vi "doDFSM_Alive.vi"(0 "HGF_DeviceBase":refnum<class "HGF_DeviceBase.lvclass">, 3 "DFSM_Internals in":T1, 5 "error in (no error)":errorcluster) -> (14 "dup HGF_DeviceBase":refnum<class "HGF_DeviceBase.lvclass">, 17 "DFSM_Internals out":T1, 19 "error out":errorcluster)   [LabVIEW 2014, in "HGF_DeviceBaseClasses.lvlib" / "HGF_DeviceBase.lvclass"]
doc: "This VI performs <B>do</B> action of DeviceFSM.Alive.\n\n<b>Hint:</b> This is a dynamic dispatch VI to be implemented by child classes."
uses:
  HGF_DeviceBase.lvclass
  HGF_StateCharts/HGF_DeviceFSM/HGF_DeviceFSM_Internals.ctl
  HGF_DeviceBaseClasses.lvlib
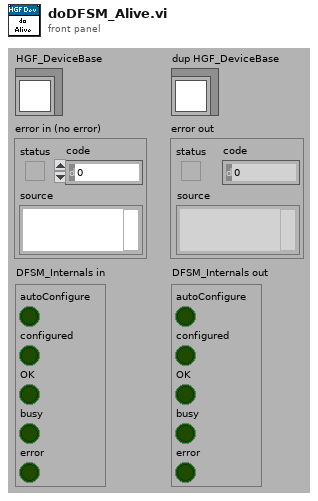
[diagram p1: front panel]
types:
  T1 = typedef "HGF_DeviceBaseClasses.lvlib/HGF_DeviceFSM_Internals.ctl" = cluster{"autoConfigure":bool, "configured":bool, "OK":bool, "busy":bool, "error":bool}
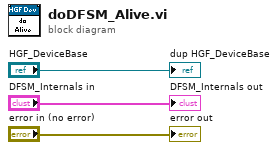
[diagram p0: block diagram]
diagram:
  "error out" <- "error in (no error)"
  "dup HGF_DeviceBase" <- "HGF_DeviceBase"
  "DFSM_Internals out" <- "DFSM_Internals in"
